vi "Test App Context of Nested App.vi"(8 "error in (no error)":errorcluster, 11 "Application Test in":refnum<class "Application Test.lvclass">) -> (0 "error out":errorcluster, 3 "Application Test out":refnum<class "Application Test.lvclass">)   [LabVIEW 2020, in "Application Test.lvclass"]
uses:
  Application Test.lvclass
  C:/Program Files (x86)/National Instruments/LabVIEW 2020/vi.lib/Asteme/LUnit/Test Case.lvclass
  Framework/Application/Application.lvclass
  C:/Users/anton/Documents/GitHub/Triarc-Framework/source/Framework/Process/Process.lvclass
  Framework/Process/Process.lvclass
  Framework/Process/Process.lvclass/Process.ctl
  Framework/Application/Application.lvclass/Application.ctl
  <vilib>/Asteme/LUnit/Test Case.lvclass/Test Case.ctl
  <vilib>/Asteme/LUnit/LUnit Assertion Result.lvclass/LUnit Assertion Result.ctl
  Framework/Application/Private/Add Process to Map.vi
  Framework/Process/Protected/Messaging/Enqueue Message.vi
  Framework/Process/Protected/SubVIs/Set Context.vi
  Framework/Process/Public/Lifecycle/Get Lifecycle State.vi
  <vilib>/Asteme/LUnit/Palette/Pass.vi
  <vilib>/Asteme/LUnit/Palette/Fail.vi
  <vilib>/Asteme/LUnit/Variant to string.vi
  <vilib>/Asteme/LUnit/Set Assertion Type.vi
  Framework/Process/Private/SubVIs/Wait for finish.vi
  Framework/Process/Private/SubVIs/Set Lifecycle State.vi
  <vilib>/Utility/error.llb/Clear Errors.vi
  Framework/Process/Community/Leave Process Loop.vi
  <vilib>/Asteme/LUnit/Add test result.vi
  <vilib>/Asteme/LUnit/LUnit Write Passed.vi
  <vilib>/Asteme/LUnit/LUnit Get Test Case.vi
  <vilib>/Asteme/LUnit/Assertion Result/LUnit Get Test Name.vi
  <vilib>/Asteme/LUnit/LUnit Write Message.vi
  <vilib>/Asteme/LUnit/LUnit Write Description.vi
  <vilib>/Asteme/LUnit/LUnit Write Assertion Type.vi
  <vilib>/Asteme/LUnit/Read Test Case Name.vi
  <vilib>/Utility/error.llb/Error Cluster From Error Code.vi
  Framework/Application/Private/Update Context for Owned Processes.vi
  <vilib>/Utility/Data Type/Get Type Information.vi
  <vilib>/Utility/LVClass/Get LV Class Name.vi
  <vilib>/Asteme/LUnit/LUnit Assertion Result.lvclass
  <vilib>/Asteme/LUnit/Test Case.lvclass
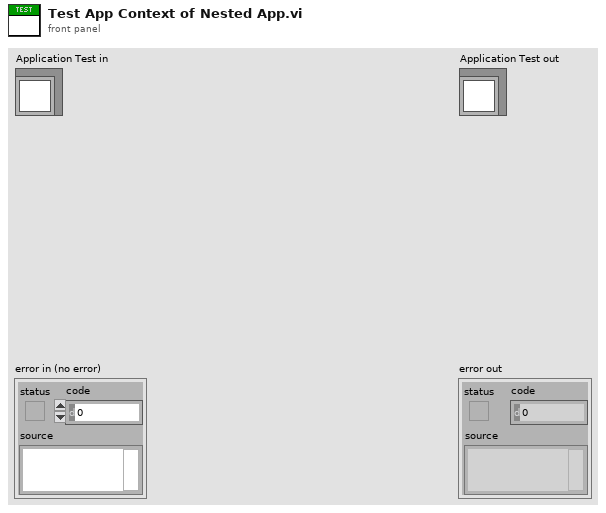
[diagram p1: front panel]
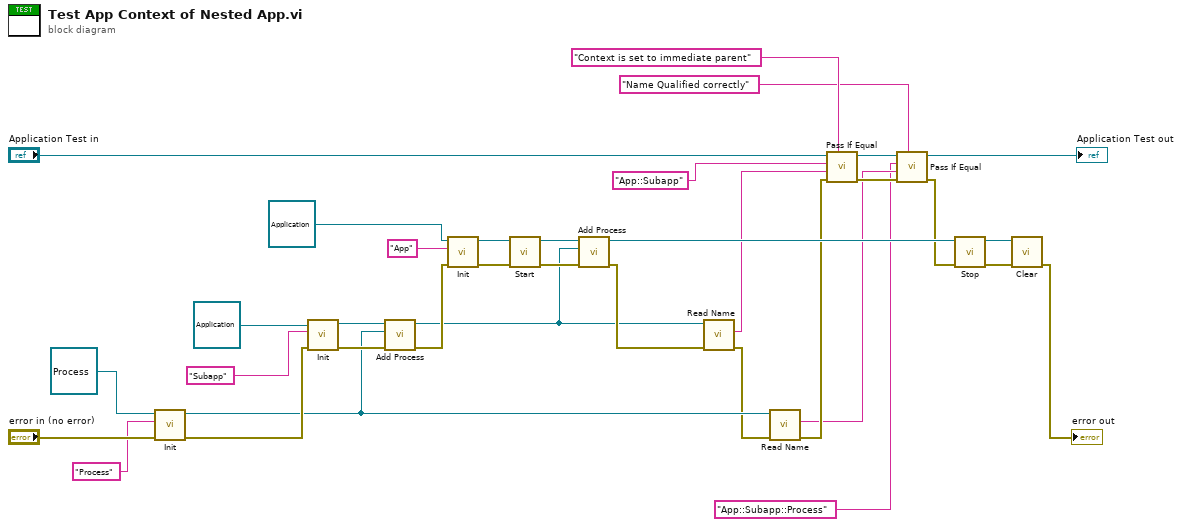
[diagram p0: block diagram]
diagram:
  n1 = call-dynamic "Init.vi"("error in (no error)"="error in (no error)", "Name"="Process", "Process In"=refnum<class "Process.lvclass"> refnum) -> ("error out"=w14:errorcluster, "Process Out"=w13:refnum<class "Process.lvclass">)  [unwired: 7 in]
  n2 = call-dynamic "Init.vi"("error in (no error)"=w14, "Name"="Subapp", "Process In"=refnum<class "Application.lvclass"> refnum ("Application.lvclass")) -> ("error out"=w19:errorcluster, "Process Out"=w20:refnum<class "Application.lvclass">)  [unwired: 7 in]
  n3 = call "Add Process.vi"("error in (no error)"=w19, "Process"=w13, "Rig In"=w20) -> ("error out"=w18:errorcluster, "Rig Out"=w1:refnum<class "Application.lvclass">)  [unwired: 7 in]
  n4 = call-dynamic "Init.vi"("error in (no error)"=w18, "Name"="App", "Process In"=refnum<class "Application.lvclass"> refnum ("Application.lvclass")) -> ("error out"=w34:errorcluster, "Process Out"=w35:refnum<class "Application.lvclass">)  [unwired: 7 in]
  n5 = call "Start.vi"("error in (no error)"=w34, "Process In"=w35) -> ("error out"=w32:errorcluster, "Process Out"=w22:refnum<class "Application.lvclass">)  [unwired: 8 in]
  n6 = call "Add Process.vi"("error in (no error)"=w32, "Process"=w1, "Rig In"=w22) -> ("error out"=w12:errorcluster, "Rig Out"=w25:refnum<class "Application.lvclass">)  [unwired: 7 in]
  n7 = call-dynamic "Read Name.vi"("error in (no error)"=w12, "Process In"=w1) -> ("error out"=w2:errorcluster, "Qualified Name"=w4:string)  [unwired: 6 in, 2 out]
  n8 = call-dynamic "Read Name.vi"("error in (no error)"=w2, "Process In"=w13) -> ("error out"=w11:errorcluster, "Qualified Name"=w7:string)  [unwired: 6 in, 2 out]
  n9 = call <vilib>:"Pass If Equal.vi"("Description"="Context is set to immediate parent", "error in (no error)"=w11, "Actual"=w4, "Expected"="App::Subapp" ("Name"), "Test Case In"="Application Test in") -> ("error out"=w9:errorcluster, "Test Case Out"=w31:refnum<class "Application Test.lvclass">)  [unwired: 5 in]
  n10 = call <vilib>:"Pass If Equal.vi"("Description"="Name Qualified correctly", "error in (no error)"=w9, "Actual"=w7, "Expected"="App::Subapp::Process" ("Name"), "Test Case In"=w31) -> ("error out"=w8:errorcluster, "Test Case Out"=→"Application Test out":refnum<class "Application Test.lvclass">)  [unwired: 5 in]
  n11 = call "Stop.vi"("error in (no error)"=w8, "Process In"=w25) -> ("error out"=w28:errorcluster, "Process Out"=w33:refnum<class "Application.lvclass">)  [unwired: 7 in, 1 out]
  n12 = call-dynamic "Clear.vi"("error in (no error)"=w28, "Application In"=w33) -> ("error out"=→"error out":errorcluster)  [unwired: 8 in, 1 out]
